vi "Check Loop Error1.vi"(8 "dup error in":errorcluster, 9 "Igonre Error":i32[](array[numeric]), 10 "Exit or Error":bool) -> (0 "Error Out":errorcluster)   [LabVIEW 2016]
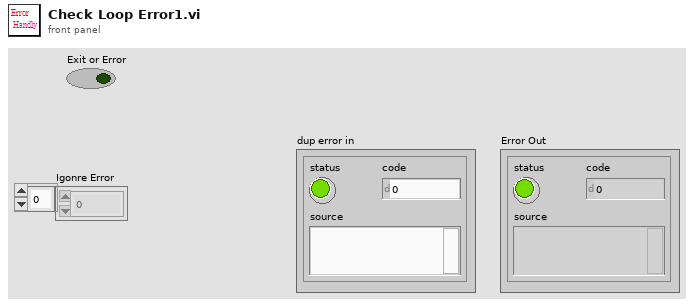
[diagram p1: front panel]
types:
  T1 = enum16{"Open", "Enqueue", "InsertQueue", "Release Queue", "Close"}
  T2 = typedef "Message Queue.lvlib/Message Cluster.ctl" = cluster{"Message":string, "Message Data":variant}
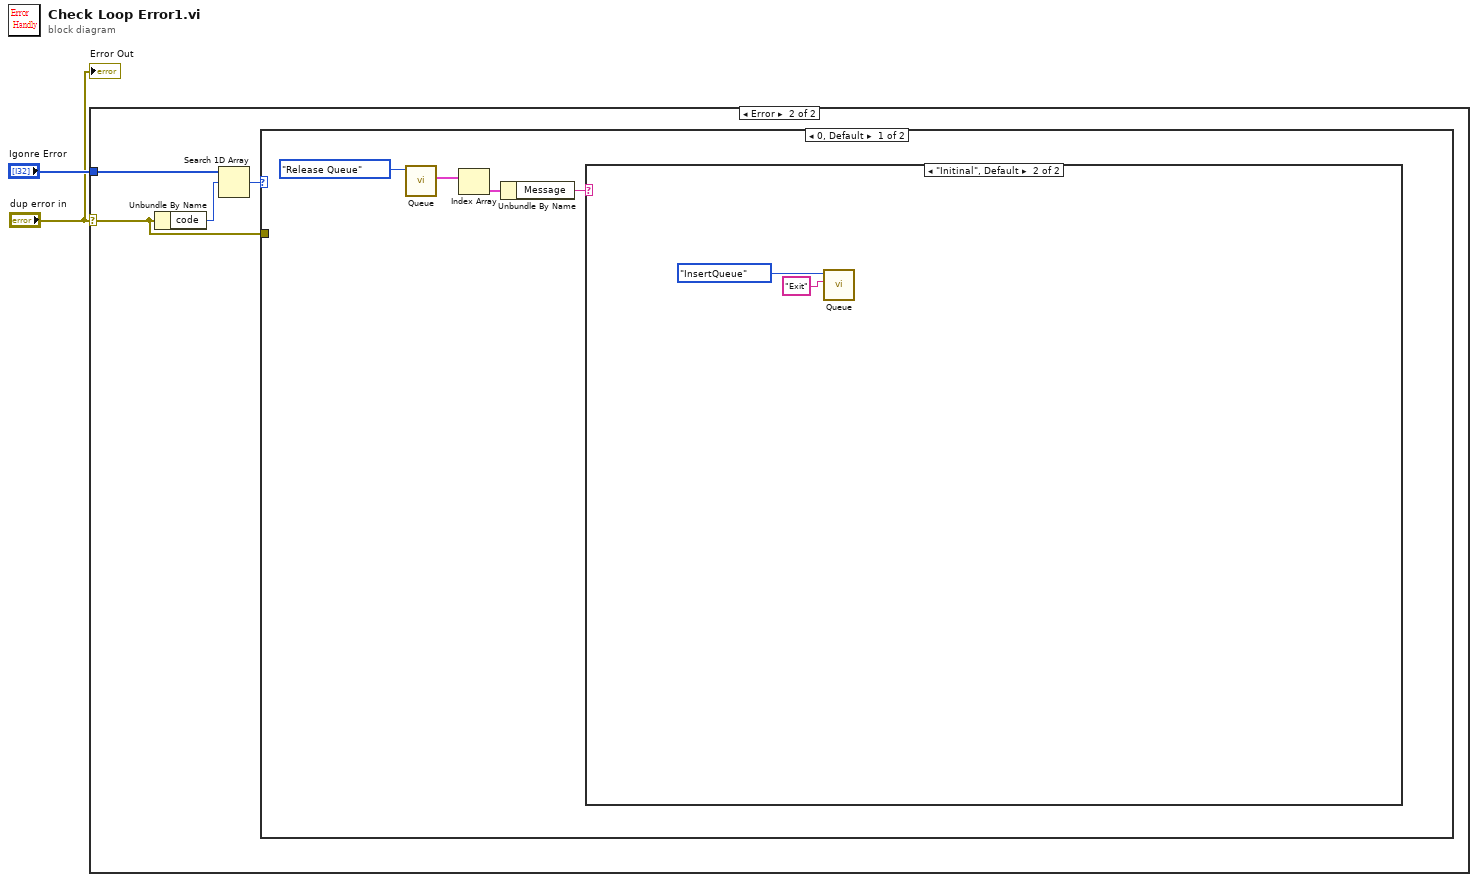
[diagram p0: block diagram]
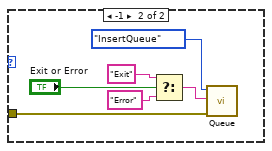
[diagram p4: hidden frame]
diagram:
  n1 = case shown="Error" "dup error in" {
    selector: "dup error in" -> [_ w3]
    tunnel: "Igonre Error" -> [_ w5]
    frame No Error {
    }
    frame Error {
      n2 = Unbundle By Name(w3) -> ("code"=w6:i32)
      n3 = Search 1D Array(1D array=w5, element=w6) -> (index of element=w4:i32)  [unwired: 1 in]
      n4 = case shown="0, Default" w4 {
        tunnel: w3 -> [_ w17]
        frame 0, Default {
          n5 = call "Queue.vi"("Function"=T1."Release Queue") -> ("Release Queue"=w9:T2[])  [unwired: 8 in, 2 out]
          n6 = Index Array(array=w9) -> (element=w8:T2)  [unwired: 1 in]
          n7 = Unbundle By Name(w8) -> ("Message"=w7:string)
          n8 = case shown="\"Initinal\", Default" w7 {
            frame "Step1" {
            }
            frame "Initinal", Default {
              n9 = call "Queue.vi"("Message"="Exit", "Function"=T1."InsertQueue") -> ()  [unwired: 7 in, 3 out]
            }
          }
        }
        frame -1 {
          n10 = Select(t="Exit" ("Message"), s="Exit or Error", f="Error" ("Message")) -> (s? t:f=w14:string)
          n11 = call "Queue.vi"("error in"=w17, "Message"=w14, "Function"=T1."InsertQueue") -> ()  [unwired: 6 in, 3 out]
        }
      }
    }
  }
  "Error Out" <- "dup error in"
